vi "PopUp_Add Language.vi"(8 "error in (no error)":errorcluster) -> (0 "error out":errorcluster, 2 "OK Pressed?":bool, 3 "NewLang Name":string)   [LabVIEW 2013, in "SET Project Editor.lvlib"]
uses:
  SET Project Editor.lvlib
  DialogEnum.ctl
panel:
  in  "Language Name":string(combo) caption="Language Name:"
  in  "Cancel":bool
  in  "OK":bool
  # "Add Language"
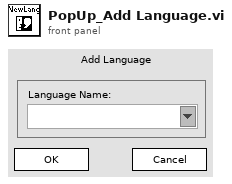
[diagram p1: front panel]
types:
  T1 = typedef "SET Project Editor.lvlib/DialogEnum.ctl" = enum16{"Idle", "Init", "Shutdown"}
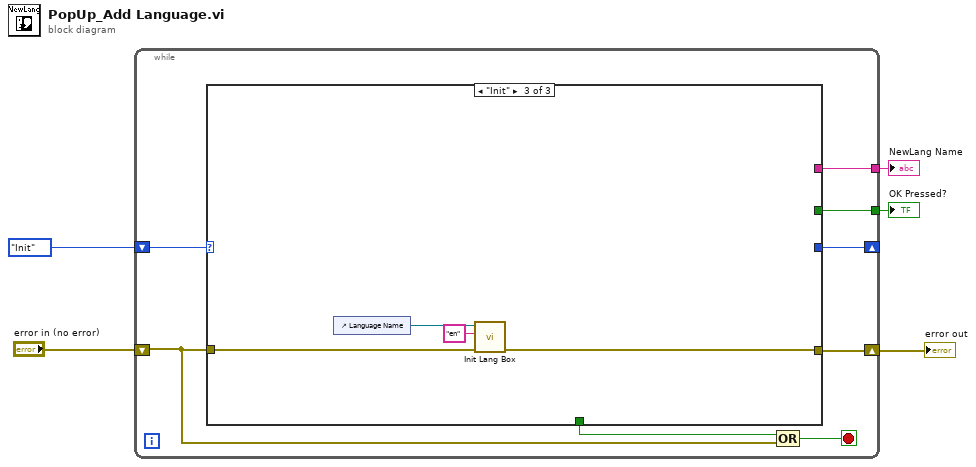
[diagram p0: block diagram]
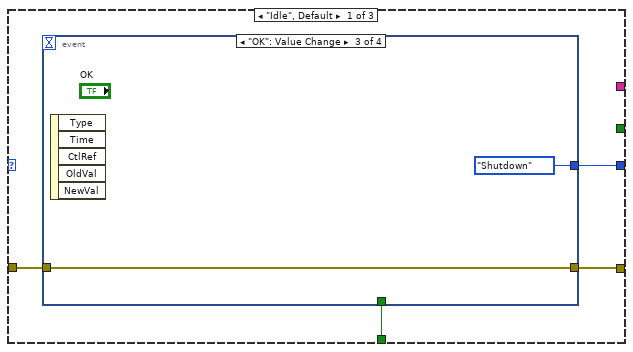
[diagram p2: hidden frame]
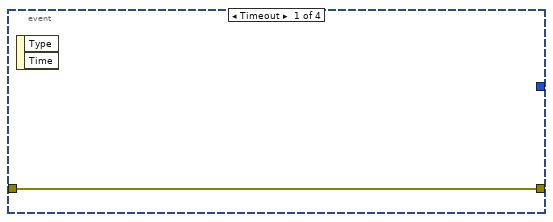
[diagram p3: hidden frame]
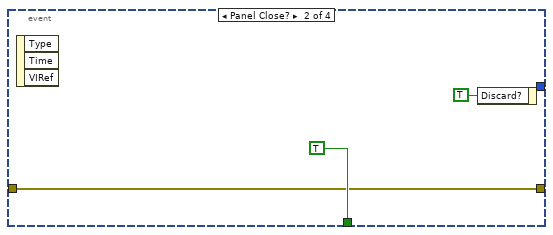
[diagram p4: hidden frame]
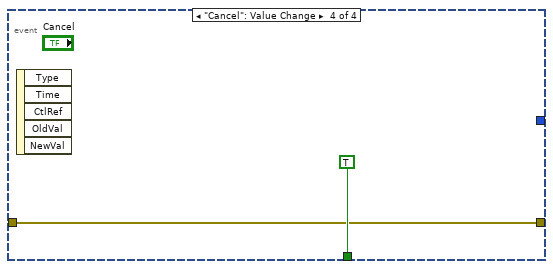
[diagram p5: hidden frame]
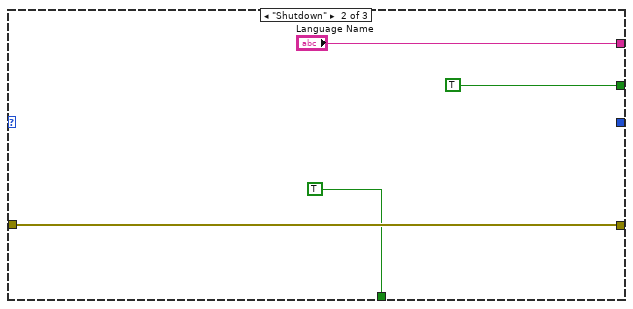
[diagram p6: hidden frame]
diagram:
  n1 = while {
    shift-right: [w12] -> w3
    shift-left: "error in (no error)" -> [w9]
    shift-right: [w11] -> _
    shift-left: DialogEnum."Init" -> [w13]
    tunnel: [w7] -> w2
    tunnel: [w6] -> w1
    stop <- w8 stop-if-true
    n2 = case shown="\"Init\"" w13 {
      tunnel: [w17 w29 w30] -> w12
      tunnel: w9 -> [w16 w29 w31]
      tunnel: [w15 TRUE _] -> w10
      tunnel: [w14 _ _] -> w11
      tunnel: [_ "Language Name" _] -> w7
      tunnel: [_ TRUE _] -> w6
      frame "Idle", Default {
        n3 = event shown="[2] \"OK\": Value Change" {
          selector: _ -> [_ _ _ _]
          dyn-events: _ -> [_ _ _ _]
          timeout: _ -> [_ _ _ _]
          tunnel: [w18 w19 w22 w24] -> w17
          tunnel: w16 -> [w18 w19 w22 w24]
          tunnel: [_ TRUE _ TRUE] -> w15
          tunnel: [_ _ DialogEnum."Shutdown" _] -> w14
          event Timeout {
            n4 = event-data() -> ()  [unwired: 1 in, 2 out]
          }
          event Panel Close? {
            n5 = event-data() -> ()  [unwired: 1 in, 3 out]
            n6 = event-data("Discard?"=TRUE) -> ()  [unwired: 1 in, 1 out]
          }
          event "OK": Value Change {
            n7 = event-data() -> ()  [unwired: 1 in, 5 out]
          }
          event "Cancel": Value Change {
            n8 = event-data() -> ()  [unwired: 1 in, 5 out]
          }
        }
      }
      frame "Shutdown" {
      }
      frame "Init" {
        n9 = control-ref of="Language Name"() -> (w33:refnum<vi>)
        n10 = call "Init Lang Box.vi"("error in (no error)"=w31, "Initial Value"="en", "ComboBox Ref in"=w33) -> ("error out"=w30:errorcluster)  [unwired: 7 in, 1 out]
      }
    }
    n11 = Compound Arithmetic op=OR(w10, w9) -> (w8:bool)
  }
  "error out" <- w3
  "NewLang Name" <- w2
  "OK Pressed?" <- w1
